vi "Spex Scan V1.00.vi"(3 "Point #":i32, 5 "Parameters":u8[](array[numeric])) -> (0 "Stop":bool, 1 "Data Out":dbl[](array[numeric]) format="%.2f")   [LabVIEW 2020]
uses:
  Globals and TypeDefs/Global Varibal Control.vi
panel:
  out "vi state":enum32{"Broken", "Idle", "Running"}(ring)
  out "window state":enum32{"Closed", "Open", "Open and Active"}(ring)
  out "Position":dbl format="%.2f"
  # "Scanning Pattern"
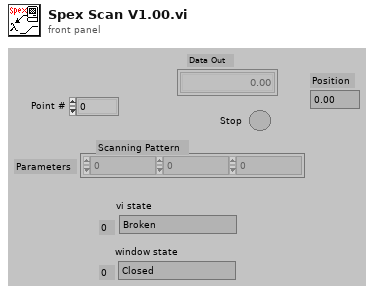
[diagram p1: front panel]
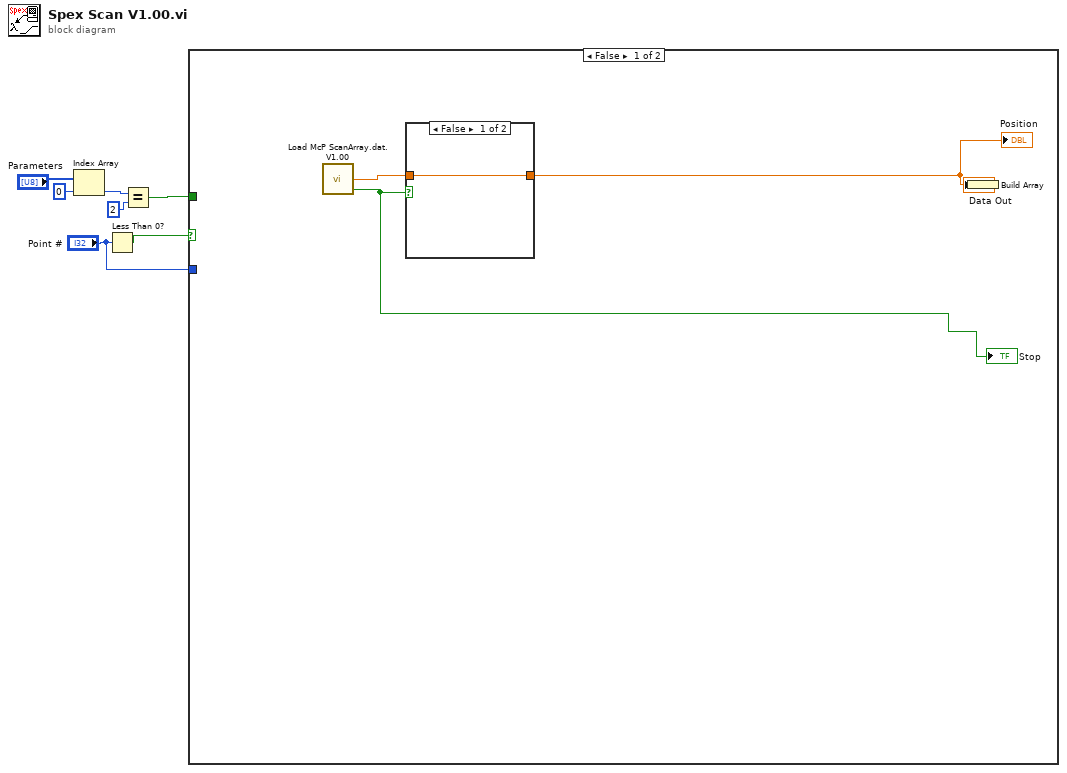
[diagram p0: block diagram]
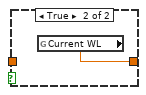
[diagram p2: hidden frame]
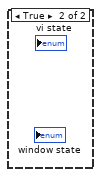
[diagram p3: hidden frame]
diagram:
  n1 = Index Array(array="Parameters", index=0 ("Index")) -> (element=w4:u8)
  n2 = Less Than 0?(x="Point #") -> (x < 0?=w7:bool)
  n3 = Equal?(x=w4, y=u8 2) -> (x = y?=w2:bool)
  n4 = case shown="False" w7 {
    tunnel: w2 -> [_ _]
    tunnel: "Point #" -> [_ _]
    frame False {
      n5 = call "Load McP ScanArray.dat.V1.00.vi"() -> ("Position"=w8:sgl, "EOF?"=w11:bool)  [unwired: 2 in, 1 out]
      "Stop" <- w11
      n6 = case shown="False" w11 {
        tunnel: w8 -> [w12 _]
        tunnel: [w12 w13] -> w9
        frame False {
        }
        frame True {
          n7 = global read "Global Varibal Control.vi" "Current WL"() -> (w13:dbl)
        }
      }
      "Position" <- w9
      n8 = Build Array(w9) -> (→"Data Out":dbl[])
    }
    frame True {
    }
  }
